vi "MecanumCode.vi"(4 "AutoCameraTrackingButton":bool, 5 "CameraAutoSpeedScaler":dbl, 6 "CamerXPosition":dbl, 7 "Max Output":dbl, 8 "robotReverse":bool, 9 "Y":dbl, 10 "X":dbl, 11 "Rotation":dbl) -> (0 "rearRight":dbl, 1 "rearLeft":dbl, 2 "frontRight":dbl, 3 "frontLeft":dbl)   [LabVIEW 2011]
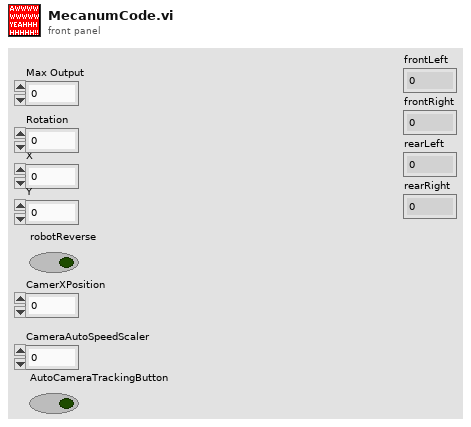
[diagram p1: front panel]
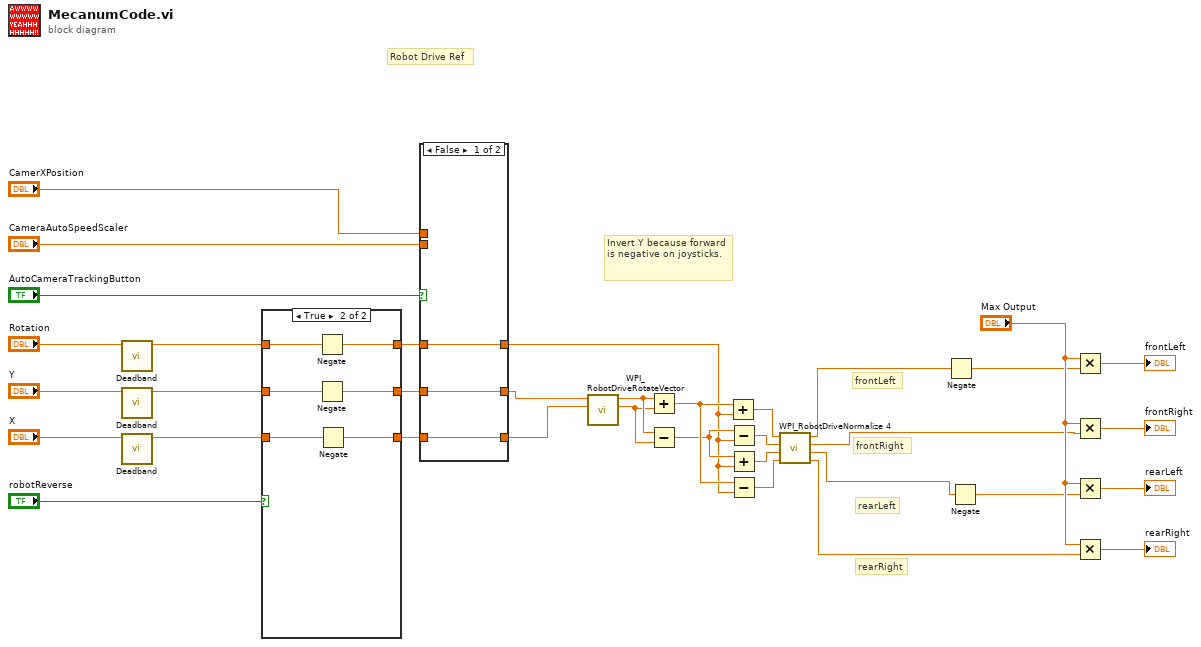
[diagram p0: block diagram]
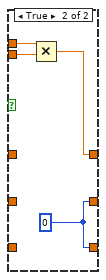
[diagram p3: hidden frame]
diagram:
  # "Invert Y because forward is negative on joysticks."
  # "rearLeft"
  # "frontRight"
  # "rearRight"
  # "frontLeft"
  # "Robot Drive Ref"
  n1 = call "Deadband.vi"("joystickValueIn"="Rotation") -> ("joystickValueOut"=w12:dbl)  [unwired: 10 in]
  n2 = call "Deadband.vi"("joystickValueIn"="Y") -> ("joystickValueOut"=w10:dbl)  [unwired: 10 in]
  n3 = call "Deadband.vi"("joystickValueIn"="X") -> ("joystickValueOut"=w8:dbl)  [unwired: 10 in]
  n4 = case shown="True" "robotReverse" {
    tunnel: [w38 w41] -> w17
    tunnel: w12 -> [w38 w44]
    tunnel: [w37 w42] -> w16
    tunnel: w10 -> [w37 w43]
    tunnel: [w36 w39] -> w15
    tunnel: w8 -> [w36 w40]
    frame False {
    }
    frame True {
      n5 = Negate(x=w44) -> (-x=w41:dbl)
      n6 = Negate(x=w43) -> (-x=w42:dbl)
      n7 = Negate(x=w40) -> (-x=w39:dbl)
    }
  }
  n8 = case shown="False" "AutoCameraTrackingButton" {
    tunnel: [w47 w48] -> w23
    tunnel: w15 -> [w47 _]
    tunnel: [w46 w48] -> w14
    tunnel: w16 -> [w46 _]
    tunnel: [w45 w49] -> w22
    tunnel: w17 -> [w45 _]
    tunnel: "CameraAutoSpeedScaler" -> [_ w50]
    tunnel: "CamerXPosition" -> [_ w51]
    frame False {
    }
    frame True {
      w48 = 0
      n9 = Multiply(x=w51, y=w50) -> (x*y=w49:dbl)
    }
  }
  n10 = call <vilib>:"WPI_RobotDriveRotateVector.vi"("X"=w23, "Y"=w14) -> ("X'"=w34:dbl, "Y'"=w35:dbl)  [unwired: 1 in, 7 out]
  n11 = Add(x=w35, y=w34) -> (x+y=w32:dbl)
  n12 = Subtract(x=w35, y=w34) -> (x-y=w30:dbl)
  n13 = Add(x=w32, y=w22) -> (x+y=w28:dbl)
  n14 = Subtract(x=w30, y=w22) -> (x-y=w29:dbl)
  n15 = Add(x=w30, y=w22) -> (x+y=w31:dbl)
  n16 = Subtract(x=w32, y=w22) -> (x-y=w33:dbl)
  n17 = call <vilib>:"WPI_RobotDriveNormalize 4.vi"("D"=w33, "C"=w31, "B"=w29, "A"=w28) -> ("D'"=w27:dbl, "C'"=w3:dbl, "B'"=w5:dbl, "A'"=w6:dbl)
  n18 = Negate(x=w6) -> (-x=w7:dbl)
  n19 = Negate(x=w3) -> (-x=w4:dbl)
  n20 = Multiply(x="Max Output", y=w7) -> (x*y=→"frontLeft":dbl)
  n21 = Multiply(x="Max Output", y=w5) -> (x*y=→"frontRight":dbl)
  n22 = Multiply(x="Max Output", y=w4) -> (x*y=→"rearLeft":dbl)
  n23 = Multiply(x="Max Output", y=w27) -> (x*y=→"rearRight":dbl)
